vi "Initialize.vi"(0 "Display State In":T3={"Current Channels Info"=[], "Help Prefix"="", "Max Display Size"=8, "Max Size"=0, "Show Buttons"=TRUE, "Data Valid"=refnum, "Show Range"=FALSE, "Range Items"=[], "Range Index"=[]}, 1 "Help Prefix":string, 2 "Max Display Size":i32=8, 3 "Range Items":string[](array[string]), 5 "Current Channels Info":T2[](array[typedef]), 6 "Range Index":i32[](array[numeric]), 7 "Previous Channels Info":T2[](array[typedef]), 9 "Container State":T4, 11 "error in (no error)":errorcluster, 12 "Show Buttons":bool=TRUE, 13 "Data Valid":T1, 14 "Show Range":bool) -> (4 "Display State Out":T3={"Current Channels Info"=[], "Help Prefix"="", "Max Display Size"=8, "Max Size"=0, "Show Buttons"=TRUE, "Data Valid"=refnum, "Show Range"=FALSE, "Range Items"=[], "Range Index"=[]}, 15 "error out":errorcluster)   [LabVIEW 2021, in "myRIO Channel List.xctl"]
doc: "The default value of the <b>Max Display Size</b> is 8.\nThe default value of the <b>Show Buttons</b> is TRUE."
uses:
  <vilib>/myRIO/Common/Express VI Framework/xctls/myRIO Channel List/myRIO Channel List.xctl
  <vilib>/_xctls/Container State.ctl
  <vilib>/myRIO/Common/Express VI Framework/xctls/myRIO Channel List/State.ctl
  <vilib>/myRIO/Common/Profile Manager Framework/typedefs/Channel Info.ctl
  <vilib>/myRIO/Common/Express VI Framework/typedefs/Data Validate Ref.ctl
  <vilib>/myRIO/Common/Express VI Framework/xctls/myRIO Channel List/Data.ctl
  <vilib>/myRIO/Common/Express VI Framework/xctls/myRIO Channel List/typedefs/Channel Data.ctl
  <vilib>/myRIO/Common/Express VI Framework/xctls/myRIO Channel List/typedefs/Remove Channel.ctl
  <vilib>/myRIO/Common/Express VI Framework/vis/Express VI Framework Strings Global.vi
  <vilib>/regexp/Match Regular Expression.xnode
  <vilib>/_xctls/XControlSupport.lvlib
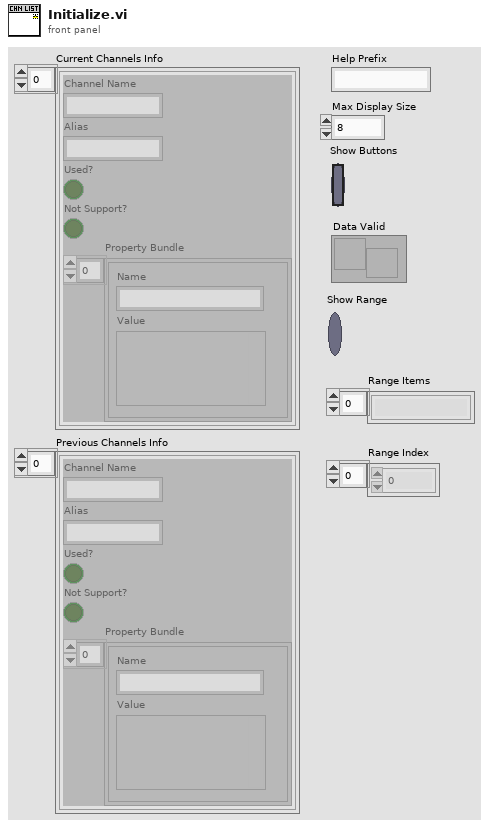
[diagram p1: front panel]
types:
  T1 = typedef "Data Validate Ref.ctl" = refnum<user-event>
  T2 = typedef "Channel Info.ctl" = cluster{"Channel Name":string, "Alias":string, "Used?":bool, "Not Support?":bool, "Property Bundle":cluster{"Name":string, "Value":variant}[]}
  T3 = typedef "myRIO Channel List.xctl/State.ctl" = cluster{"Current Channels Info":T2[], "Help Prefix":string, "Max Display Size":i32, "Max Size":i32, "Show Buttons":bool, "Data Valid":T1, "Show Range":bool, "Range Items":string[], "Range Index":i32[]}
  T4 = typedef "XControlSupport.lvlib/Container State.ctl" = cluster{"Indicator?":bool, "Run Mode?":bool, " Refnum":refnum<vi>}
  T5 = typedef "myRIO Channel List.xctl/Data.ctl" = T6[]
  T6 = typedef "myRIO Channel List.xctl/Channel Data.ctl" = cluster{"Channel Name":u16, "Channel Alias":string, "Remove Channel":T7, "Index":i32}
  T7 = typedef "myRIO Channel List.xctl/Remove Channel.ctl" = bool
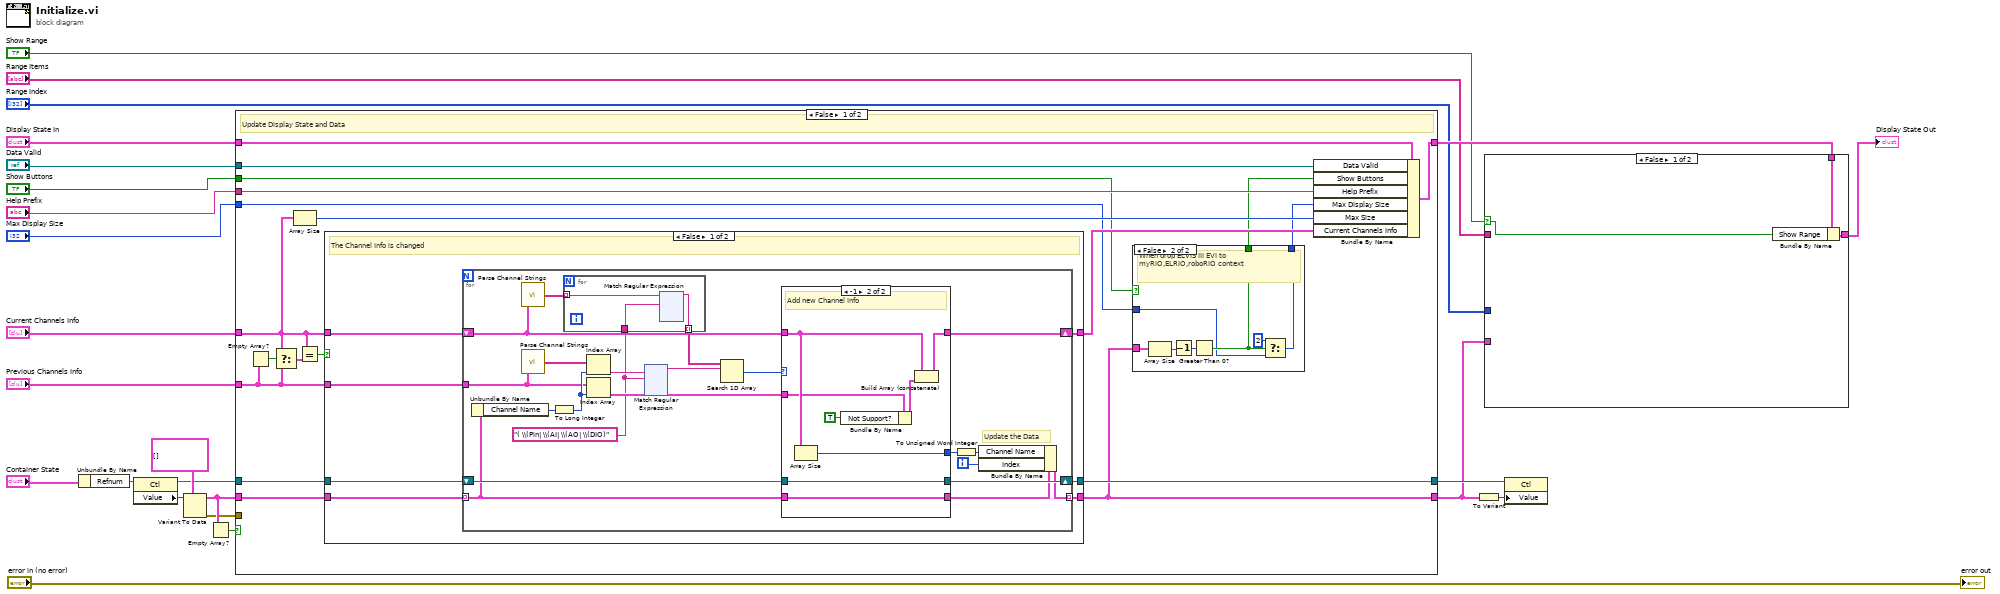
[diagram p0: block diagram]
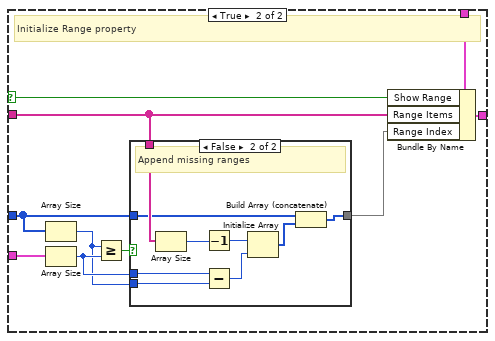
[diagram p2: hidden frame]
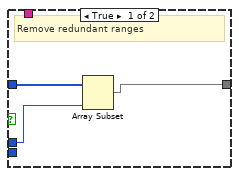
[diagram p3: hidden frame]
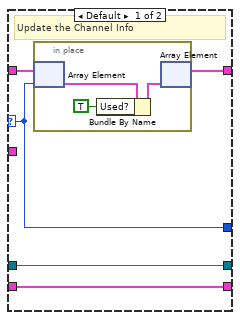
[diagram p5: hidden frame]
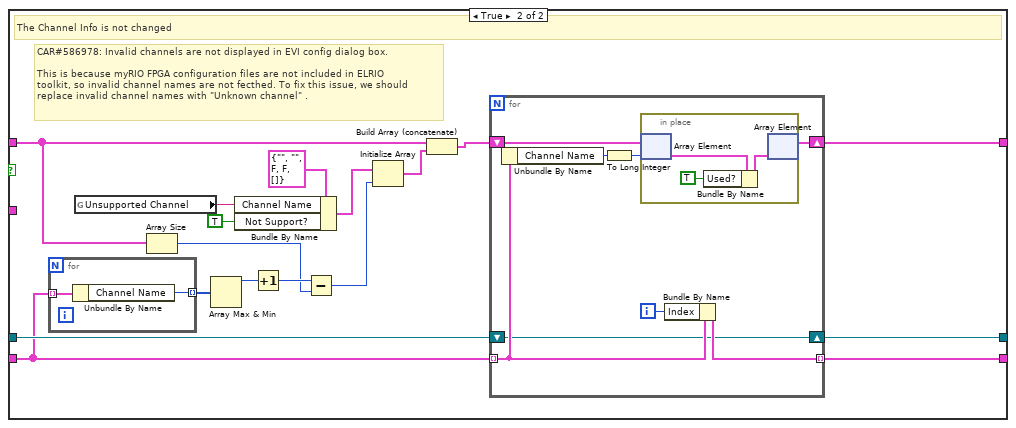
[diagram p6: hidden frame]
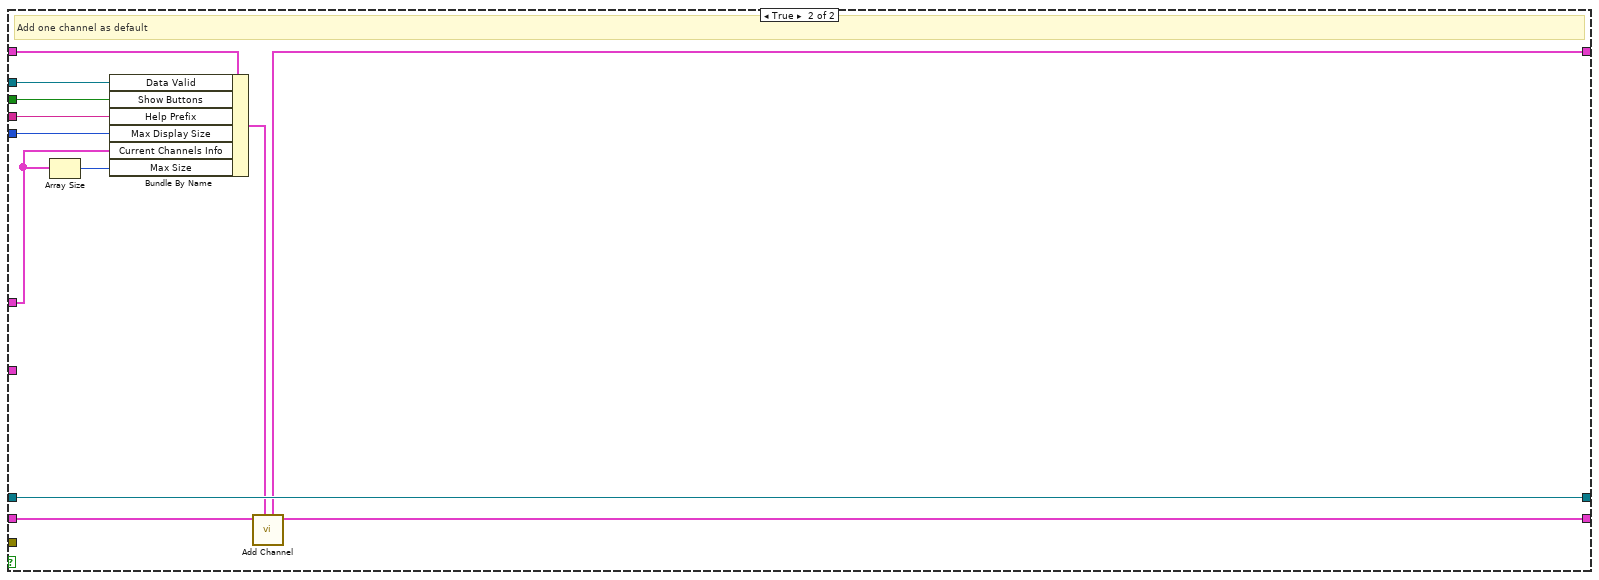
[diagram p7: hidden frame]
diagram:
  n1 = Unbundle By Name("Container State") -> ("Refnum"=w22:refnum<vi>)
  n2 = property class="Ctl"(reference=w22) -> (reference out=w16:refnum<vi>, "Value"=w21:variant)  [unwired: 1 in, 1 out]
  n3 = Variant To Data(type=T5 [] ("Channel List"), Variant=w21) -> (data=w18:T5, error out=w14:errorcluster)  [unwired: 1 in]
  n4 = Empty Array?(array=w18) -> (empty?=w19:bool)
  n5 = case shown="False" w19 {
    tunnel: w18 -> [w39 w375]
    tunnel: "Current Channels Info" -> [w34 w368]
    tunnel: w16 -> [w38 w374]
    tunnel: "Previous Channels Info" -> [w40 _]
    tunnel: w14 -> [_ _]
    tunnel: [w37 w374] -> w13
    tunnel: [w28 w366] -> w5
    tunnel: "Max Display Size" -> [w26 w373]
    tunnel: "Help Prefix" -> [w36 w372]
    tunnel: "Display State In" -> [w31 w371]
    tunnel: [w32 w367] -> w6
    tunnel: "Show Buttons" -> [w29 w365]
    tunnel: "Data Valid" -> [w33 w364]
    frame False {
      # "Update Display State and Data"
      n6 = Empty Array?(array=w40) -> (empty?=w43:bool)
      n7 = Select(t=w34, s=w43, f=w40) -> (s? t:f=w42:T2[])
      n8 = Array Size(array=w34) -> (size(s)=w35:i32)
      n9 = Equal?(x=w34, y=w42) -> (x = y?=w41:bool)
      n10 = case shown="False" w41 {
        tunnel: w34 -> [w57 w341]
        tunnel: [w55 w350] -> w30
        tunnel: w40 -> [w58 _]
        tunnel: w39 -> [w59 w346]
        tunnel: w38 -> [w56 w348]
        tunnel: [w54 w347] -> w37
        tunnel: [w53 w349] -> w28
        frame False {
          # "The Channel Info is changed"
          n11 = for {
            tunnel: w59 -> [w78] mode=indexing
            tunnel: w58 -> [w65]
            tunnel: [w73] -> w53 mode=indexing
            shift-right: [w76] -> w54
            shift-left: w56 -> [w79]
            shift-right: [w75] -> w55
            shift-left: w57 -> [w68]
            i -> [w70]
            w60 = "( \\(Pin| \\(AI| \\(AO| \\(DIO)" ("regular expression")
            # "Update the Data"
            n12 = Unbundle By Name(w78) -> ("Channel Name"=w80:u16)
            n13 = call <vilib>:"Parse Channel Strings.vi"("Channels Info"=w68) -> ("Channel Strings"=w63:string[])
            n14 = call <vilib>:"Parse Channel Strings.vi"("Channels Info"=w65) -> ("Channel Strings"=w67:string[])
            n15 = To Long Integer(number=w80) -> (32bit integer=w66:i32)
            n16 = for {
              tunnel: w63 -> [w199] mode=indexing
              tunnel: [w200] -> w62 mode=indexing
              tunnel: w60 -> [w198]
              n17 = xnode "Match Regular Expression"("input string"=w199, "regular expression"=w198) -> ("before match"=w200:string)  [unwired: 4 in, 4 out]
            }
            n18 = Index Array(array=w67, index=w66) -> (element=w61:string)
            n19 = Index Array(array=w65, index=w66) -> (element=w74:T2)
            n20 = xnode "Match Regular Expression"("input string"=w61, "regular expression"=w60) -> ("before match"=w64:string)  [unwired: 4 in, 4 out]
            n21 = Search 1D Array(1D array=w62, element=w64) -> (index of element=w77:i32)  [unwired: 1 in]
            n22 = case shown="-1" w77 {
              selector: w77 -> [w318 _]
              tunnel: w79 -> [w322 w333]
              tunnel: w78 -> [w321 w327]
              tunnel: [w321 w327] -> w72
              tunnel: w68 -> [w319 w332]
              tunnel: [w322 w333] -> w76
              tunnel: [w320 w331] -> w75
              tunnel: w74 -> [_ w330]
              tunnel: [w318 w326] -> w71
              frame Default {
                # "Update the Channel Info"
                n23 = in-place {
                  n24 = in-place-array #1(w319, w318) -> (w324:T2)
                  n25 = Bundle By Name(cluster=w324, "Used?"=TRUE) -> (w323:T2)
                  n26 = in-place-array #1(w323) -> (w320:T2[])  [unwired: 1 out]
                }
              }
              frame -1 {
                # "Add new Channel Info"
                n27 = Array Size(array=w332) -> (size(s)=w326:i32)
                n28 = Bundle By Name(cluster=w330, "Not Support?"=TRUE) -> (w329:T2)
                n29 = Build Array (concatenate)(w332, w329) -> (w331:T2[])
              }
            }
            n30 = To Unsigned Word Integer(number=w71) -> (unsigned 16bit integer=w69:u16)
            n31 = Bundle By Name(cluster=w72, "Channel Name"=w69, "Index"=w70) -> (w73:T6)
          }
        }
        frame True {
          # "CAR#586978: Invalid channels are not displayed in EVI config dialog box.\n\nThis is because myRIO FPGA configuration files are not included in ELRIO\ntoolkit, so invalid channel names are not fecthed. To fix this issue, we should \nreplace invalid channel names with \"Unknown channel\" ."
          # "The Channel Info is not changed"
          n32 = for {
            tunnel: w346 -> [w352] mode=indexing
            tunnel: [w351] -> w345 mode=indexing
            n33 = Unbundle By Name(w352) -> ("Channel Name"=w351:u16)
          }
          n34 = global read "Express VI Framework Strings Global.vi" "Unsupported Channel"() -> (w334:string)
          n35 = Array Size(array=w341) -> (size(s)=w343:i32)
          n36 = Array Max & Min(array=w345) -> (max value=w338:u16)  [unwired: 3 out]
          n37 = Bundle By Name(cluster=T2 {"Channel Name"="", "Alias"="", "Used?"=FALSE, "Not Support?"=FALSE, "Property Bundle"=[]} ("element"), "Channel Name"=w334, "Not Support?"=TRUE) -> (w335:T2)
          n38 = Increment(x=w338) -> (x+1=w344:u16)
          n39 = Subtract(x=w344, y=w343) -> (x-y=w342:i32)
          n40 = Initialize Array(w335, w342) -> (w340:T2[])
          n41 = Build Array (concatenate)(w341, w340) -> (w339:T2[])
          n42 = for {
            shift-right: [w358] -> w350
            shift-left: w339 -> [w360]
            tunnel: w346 -> [w357] mode=indexing
            tunnel: [w356] -> w349 mode=indexing
            shift-right: [w354] -> w347
            shift-left: w348 -> [w354]
            i -> [w355]
            n43 = Unbundle By Name(w357) -> ("Channel Name"=w359:u16)
            n44 = To Long Integer(number=w359) -> (32bit integer=w353:i32)
            n45 = in-place {
              n46 = in-place-array #2(w360, w353) -> (w363:T2)
              n47 = Bundle By Name(cluster=w363, "Used?"=TRUE) -> (w361:T2)
              n48 = in-place-array #2(w361) -> (w358:T2[])  [unwired: 1 out]
            }
            n49 = Bundle By Name(cluster=w357, "Index"=w355) -> (w356:T6)
          }
        }
      }
      n50 = case shown="False" w29 {
        selector: w29 -> [w45 _]
        tunnel: w28 -> [_ w52]
        tunnel: [w45 w49] -> w27
        tunnel: w26 -> [w44 w46]
        tunnel: [w44 w47] -> w25
        frame True {
        }
        frame False {
          # "When drop ELVIS III EVI to myRIO,ELRIO,roboRIO context"
          n51 = Array Size(array=w52) -> (size(s)=w51:i32)
          n52 = Decrement(x=w51) -> (x-1=w50:i32)
          n53 = Greater Than 0?(x=w50) -> (x > 0?=w49:bool)
          n54 = Select(t=2 ("Max Display Size"), s=w49, f=w46) -> (s? t:f=w47:i32)
        }
      }
      n55 = Bundle By Name(cluster=w31, "Data Valid"=w33, "Show Buttons"=w27, "Help Prefix"=w36, "Max Display Size"=w25, "Max Size"=w35, "Current Channels Info"=w30) -> (w32:T3)
    }
    frame True {
      # "Add one channel as default"
      n56 = Array Size(array=w368) -> (size(s)=w369:i32)
      n57 = Bundle By Name(cluster=w371, "Data Valid"=w364, "Show Buttons"=w365, "Help Prefix"=w372, "Max Display Size"=w373, "Current Channels Info"=w368, "Max Size"=w369) -> (w370:T3)
      n58 = call <vilib>:"Add Channel.vi"("Display State In"=w370, "Channels In"=w375) -> ("Channels Out"=w366:T5, "Display State Out"=w367:T3)  [unwired: 8 in]
    }
  }
  n59 = To Variant(anything=w5) -> (Variant=w9:variant)
  n60 = case shown="False" "Show Range" {
    selector: "Show Range" -> [w378 w379]
    tunnel: w6 -> [w377 w387]
    tunnel: w5 -> [_ w385]
    tunnel: "Range Items" -> [_ w380]
    tunnel: [w376 w382] -> w3
    tunnel: "Range Index" -> [_ w381]
    frame False {
      n61 = Bundle By Name(cluster=w377, "Show Range"=w378) -> (w376:T3)
    }
    frame True {
      # "Initialize Range property"
      n62 = Array Size(array=w381) -> (size(s)=w384:i32)
      n63 = Array Size(array=w385) -> (size(s)=w388:i32)
      n64 = Greater Or Equal?(x=w384, y=w388) -> (x >= y?=w383:bool)
      n65 = case shown="False" w383 {
        tunnel: [w389 w393] -> w386
        tunnel: w380 -> [_ w400]
        tunnel: w388 -> [w391 w397]
        tunnel: w384 -> [_ w396]
        tunnel: w381 -> [w390 w392]
        frame True {
          # "Remove redundant ranges"
          n66 = Array Subset(array=w390, length=w391) -> (w389:i32[])  [unwired: 1 in]
        }
        frame False {
          # "Append missing ranges"
          n67 = Array Size(array=w400) -> (size(s)=w399:i32)
          n68 = Decrement(x=w399) -> (x-1=w398:i32)
          n69 = Subtract(x=w397, y=w396) -> (x-y=w395:i32)
          n70 = Initialize Array(w398, w395) -> (w394:i32[])
          n71 = Build Array (concatenate)(w392, w394) -> (w393:i32[])
        }
      }
      n72 = Bundle By Name(cluster=w387, "Show Range"=w379, "Range Items"=w380, "Range Index"=w386) -> (w382:T3)
    }
  }
  "Display State Out" <- w3
  n73 = property class="Ctl"(reference=w13, "Value"=w9) -> ()  [unwired: 1 in, 2 out]
  "error out" <- "error in (no error)"
